vi "Set Pulse Voltage [PSV].vi"(7 "Micropulse # In":i32, 8 "error in (no error)":errorcluster, 9 "Voltage":T1, 10 "Channel Number":u32 caption="Channel Number (MP5 ONLY)") -> (0 "error out":errorcluster, 5 "Micropulse # Out":i32)   [LabVIEW 2026, in "MicroPulse_Driver.lvlib"]
doc: "Selects the voltage required for the pulsers on an individual channel basis. The default is all channels set to 300 volts.\n\nParameters:\n<channel> : MicroPulse channel. 0 = for all channels.\n<value> : Pulser voltage required, settings are: 50, 100, 150, 200, 250 and 300 volts.\n\nExample:\nPSV 4 200 : Sets channel 4 to a 200-volt pulser.\n\nSystem Compatibility:\nIndependent control of each channel’s pulser voltage is only available on MicroPulse 5. On a system where a global supply is used, a channel pulser voltage value is applied to all channels."
uses:
  MicroPulse_Driver.lvlib
  <instrlib>/MicroPulse/Public/Data/Datatypes/MP - pulser voltage.ctl
  Private/MP-Registry Action-Enum.ctl
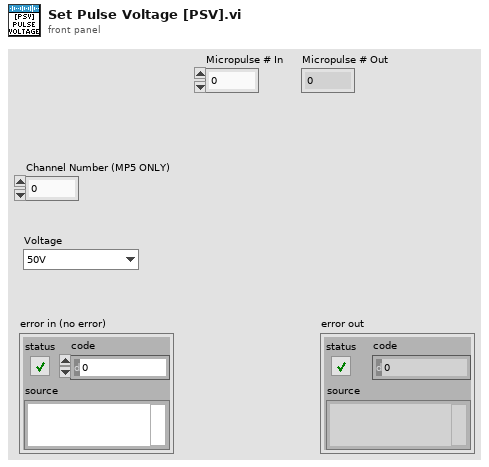
[diagram p1: front panel]
types:
  T1 = typedef "MicroPulse_Driver.lvlib/MP - pulser voltage.ctl" = enum16{"50V", "100V", "150V", "200V", "250V", "300V"}
  T2 = typedef "MicroPulse_Driver.lvlib/MP-Registry Action-Enum.ctl" = enum16{"Read", "Add Test", "Add Command", "Add Gate Command", "Add Encoder Command", "Clear Command  List", "Set Registry", "Set System Details", "Set DOF", "Set Velocity", "Disable Asynch Reads", "Enable Asynch Reads", "Add Connection", "Disconnect", "Shutdown"}
  T3 = typedef "MicroPulse_Driver.lvlib/TCP config.ctl" = cluster{"Connection ID":refnum<k5>, "IP address":string, "host port":u16, "OC timeout":i32, "Read timeout":i32, "Write timeout":i32}
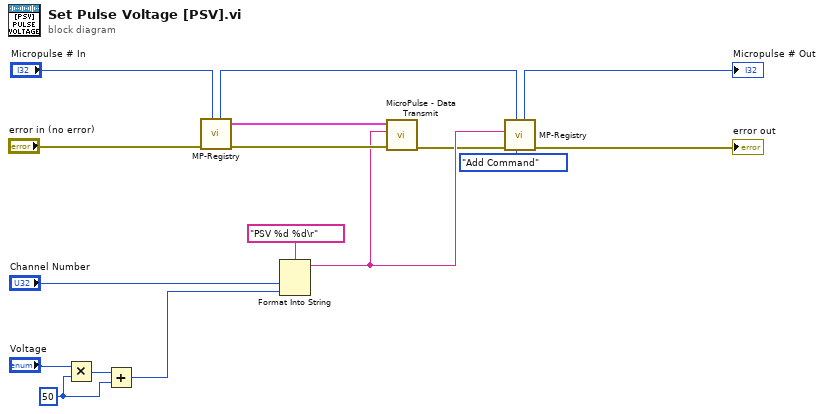
[diagram p0: block diagram]
diagram:
  w2 = 50
  n1 = Multiply(x="Voltage", y=w2) -> (x*y=w3:i32)
  n2 = Add(x=w3, y=w2) -> (x+y=w1:i32)
  n3 = call "MP-Registry.vi"("Micropulse # In"="Micropulse # In", "error in (no error)"="error in (no error)") -> ("error out"=w14:errorcluster, "TCP config"=w13:T3, "Micropulse # Out"=w8:i32)  [unwired: 6 in, 1 out]
  n4 = Format Into String(format string="PSV %d %d\r", "Channel Number", w1) -> (resulting string=w12:string)  [unwired: 2 in, 1 out]
  n5 = call "MicroPulse - Data Transmit.vi"("error in (no error)"=w14, "data"=w12, "TCP config"=w13) -> ("error out"=w10:errorcluster)  [unwired: 6 in, 2 out]
  n6 = call "MP-Registry.vi"("Action"=MP-Registry_Action-Enum."Add Command", "Micropulse # In"=w8, "error in (no error)"=w10, "Data in"=w12) -> ("error out"=→"error out":errorcluster, "Micropulse # Out"=→"Micropulse # Out":i32)  [unwired: 4 in, 2 out]
